vi "Initialize.vi"(8 "error in":errorcluster, 11 "Tacmina Settings in":T1) -> (0 "error out":errorcluster, 1 "Initialized":bool, 3 "Tacmina Settings out":T1)   [LabVIEW 2018, in "Tacmina QI.lvlib"]
uses:
  Tacmina QI.lvlib
  Tacmina QI DAQ Setting.ctl
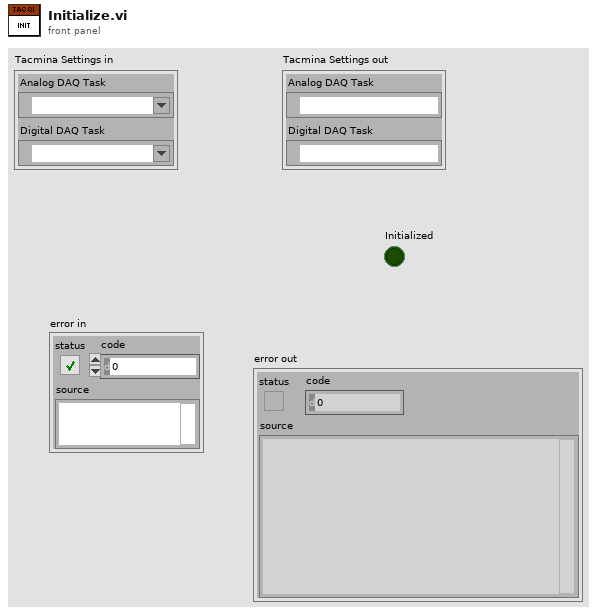
[diagram p1: front panel]
types:
  T1 = typedef "Tacmina QI.lvlib/Tacmina QI DAQ Setting.ctl" = cluster{"Analog DAQ Task":refnum<k21>, "Digital DAQ Task":refnum<k21>}
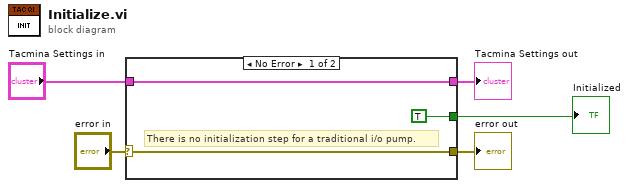
[diagram p0: block diagram]
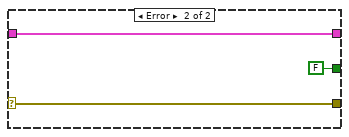
[diagram p2: hidden frame]
diagram:
  n1 = case shown="No Error" "error in" {
    selector: "error in" -> [w8 w10]
    tunnel: [w8 w10] -> w4
    tunnel: "Tacmina Settings in" -> [w7 w11]
    tunnel: [w7 w11] -> w2
    tunnel: [TRUE ("Initialized") FALSE ("Initialized")] -> w1
    frame No Error {
      # "There is no initialization step for a traditional i/o pump."
    }
    frame Error {
    }
  }
  "error out" <- w4
  "Tacmina Settings out" <- w2
  "Initialized" <- w1
